vi "verticalmenu.vi"() -> ()   [LabVIEW 2011]
uses:
  GlobalVi.vi
  GlobalPath.vi
panel:
  in  "STOP":bool
  in  "CheckPress":bool
  in  "CheckAmbient":bool
  in  "StartPress":bool
  in  "StartPanel":bool
  in  "CheckLogFile":bool
  in  "StartAmbient":bool
  # "MM Pavia"
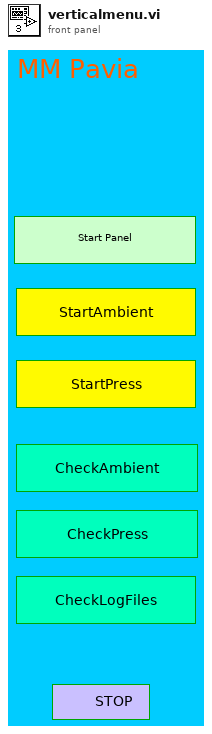
[diagram p1: front panel]
types:
  T1 = cluster{"top":i32, "left":i32, "bottom":i32, "right":i32}
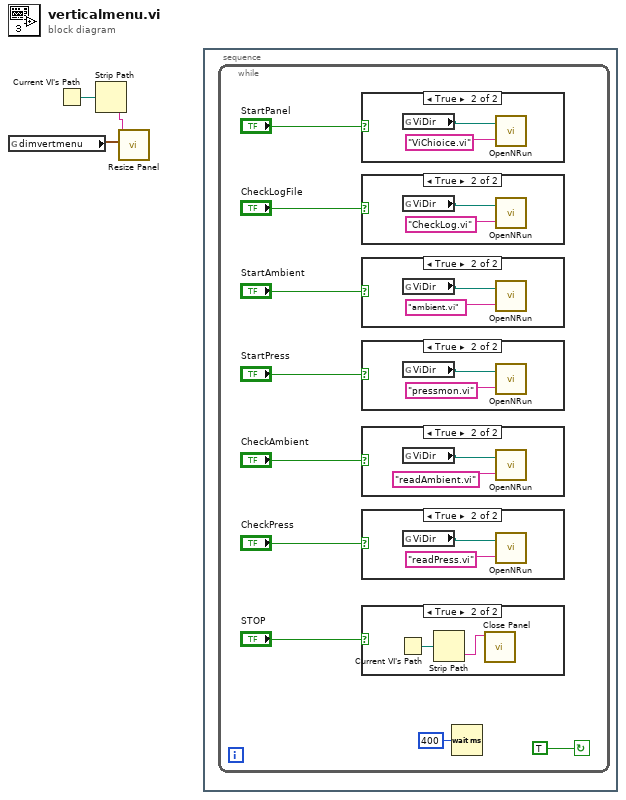
[diagram p0: block diagram]
diagram:
  n1 = global read "GlobalVi.vi" "dimvertmenu"() -> (w1:T1)
  n2 = Current VI's Path() -> (path=w3:path)
  n3 = Strip Path(path=w3) -> (name=w2:string)  [unwired: 1 out]
  n4 = call <vilib>:"Resize Panel.vi"("panel location and size"=w1, "VI name"=w2) -> ()  [unwired: 9 in, 1 out]
  n5 = stacked-sequence {
    frame #0 {
      n6 = while {
        stop <- TRUE continue-if-true
        n7 = case shown="True" "StartPanel" {
          frame False {
          }
          frame True {
            n8 = global read "GlobalPath.vi" "ViDir"() -> (w26:path)
            n9 = call "OpenNRun.vi"("VI name"="ViChioice.vi", "ViDirPath"=w26) -> ()  [unwired: 1 out]
          }
        }
        n10 = case shown="True" "CheckLogFile" {
          frame False {
          }
          frame True {
            n11 = global read "GlobalPath.vi" "ViDir"() -> (w24:path)
            n12 = call "OpenNRun.vi"("VI name"="CheckLog.vi", "ViDirPath"=w24) -> ()  [unwired: 1 out]
          }
        }
        n13 = case shown="True" "StartAmbient" {
          frame False {
          }
          frame True {
            n14 = global read "GlobalPath.vi" "ViDir"() -> (w22:path)
            n15 = call "OpenNRun.vi"("VI name"="ambient.vi", "ViDirPath"=w22) -> ()  [unwired: 1 out]
          }
        }
        n16 = case shown="True" "StartPress" {
          frame False {
          }
          frame True {
            n17 = global read "GlobalPath.vi" "ViDir"() -> (w20:path)
            n18 = call "OpenNRun.vi"("VI name"="pressmon.vi", "ViDirPath"=w20) -> ()  [unwired: 1 out]
          }
        }
        n19 = case shown="True" "CheckAmbient" {
          frame False {
          }
          frame True {
            n20 = global read "GlobalPath.vi" "ViDir"() -> (w18:path)
            n21 = call "OpenNRun.vi"("VI name"="readAmbient.vi", "ViDirPath"=w18) -> ()  [unwired: 1 out]
          }
        }
        n22 = case shown="True" "CheckPress" {
          frame False {
          }
          frame True {
            n23 = global read "GlobalPath.vi" "ViDir"() -> (w16:path)
            n24 = call "OpenNRun.vi"("VI name"="readPress.vi", "ViDirPath"=w16) -> ()  [unwired: 1 out]
          }
        }
        n25 = case shown="True" "STOP" {
          frame False {
          }
          frame True {
            n26 = Current VI's Path() -> (path=w13:path)
            n27 = Strip Path(path=w13) -> (name=w14:string)  [unwired: 1 out]
            n28 = call <vilib>:"Close Panel.vi"("VI name"=w14) -> ()  [unwired: 10 in, 1 out]
          }
        }
        n29 = Wait (ms)(milliseconds to wait=u32 400 ("millisecond multiple")) -> ()  [unwired: 1 out]
      }
    }
  }
